vi "Get Products.vi"(8 "error in (no error) 5":errorcluster, 11 "Module Number  2":dbl=1.0) -> (0 "error out 2":errorcluster, 3 "subarray":string[](array[string]))   [LabVIEW 2015, in "Copy of Untitled Library 1.lvlib"]
uses:
  Copy of Untitled Library 1.lvlib
  Controls/Enum Constant.ctl
  <userlib>/origin_lib_main/db_interface/DB Operations Enum.ctl
  <vilib>/addons/database/_DB Variant To Data/Database Variant To Data.xnode
  <userlib>/origin_lib_main/db_interface/DB Interface.lvlib
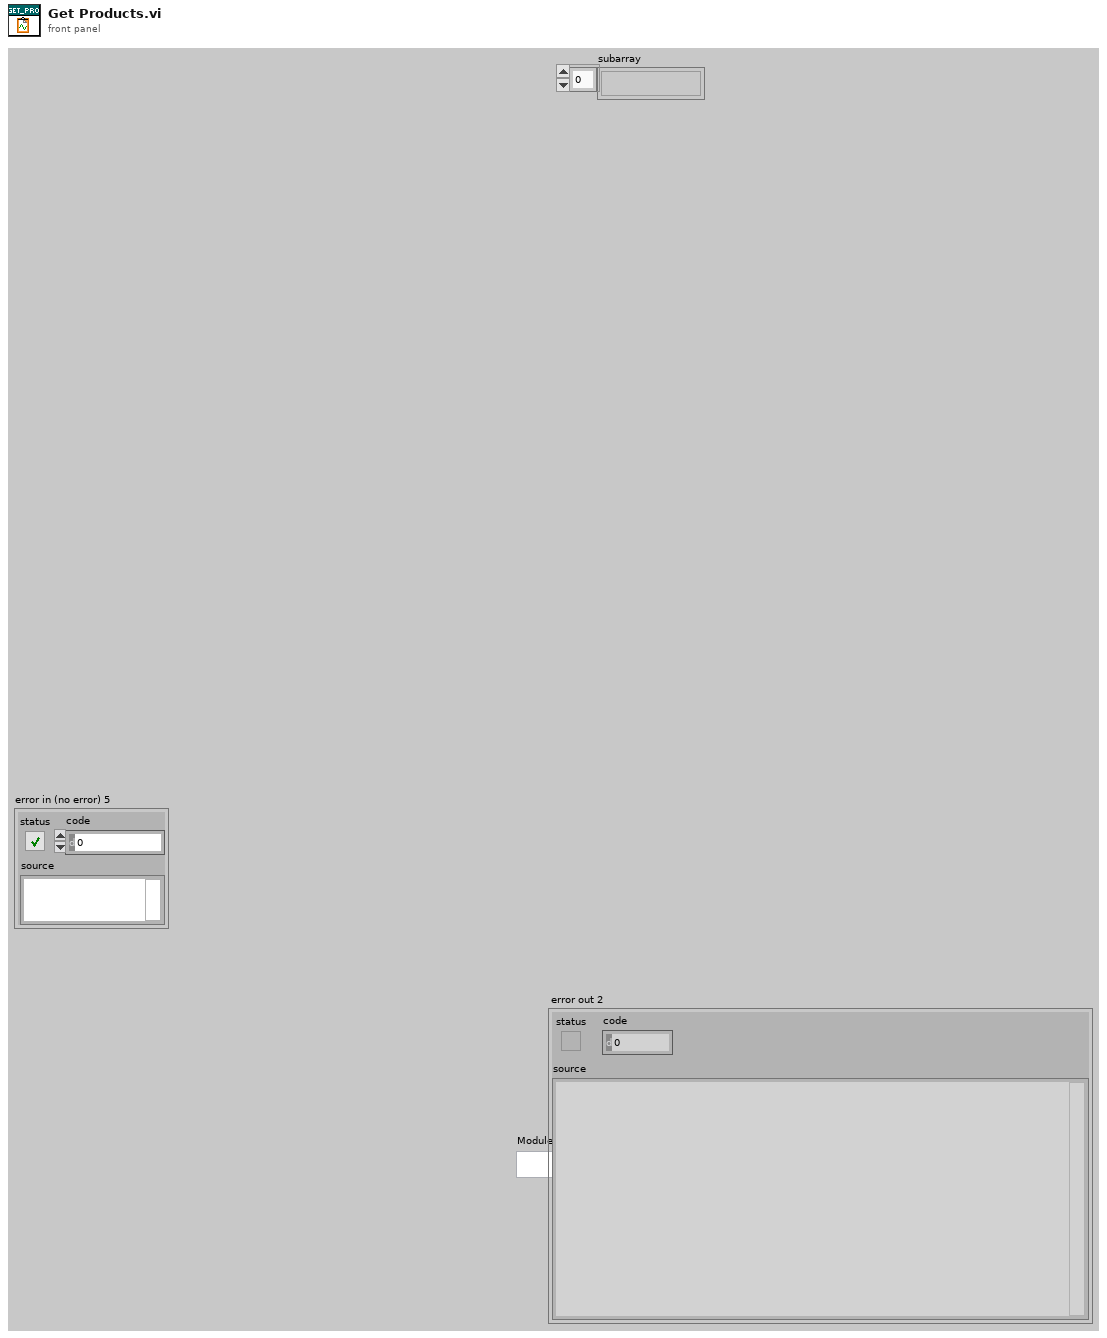
[diagram p1: front panel]
types:
  T1 = typedef "DB Interface.lvlib/DB Operations Enum.ctl" = enum16{"Select", "Update", "Insert", "Delete", "Fetch SQL Query", "Execute SQL Query", "Drop Table", "List Tables"}
  T2 = typedef "Enum Constant.ctl" = enum16{"Init", "Read", "Write"}
  T3 = typedef "FGV Data.ctl" = T4[]
  T4 = typedef "FGV Cluster Data.ctl" = cluster{"Manual/Automatic":bool, "UI Controllers ":string[], "UI Primery Key ":dbl[], "Caller Queue & MSG":T5, "Module ID":dbl, "DB Reference In":T6, "Products Columns":string[], "Cluster":cluster{"Delete Product":enum8{"Enabled", "Disabled", "Disabled and Grayed Out"}, "Add Product ":enum8{"Enabled", "Disabled", "Disabled and Grayed Out"}, "EDIT BATCH":enum8{"Enabled", "Disabled", "Disabled and Grayed Out"}, "Open Batch ":enum8{"Enabled", "Disabled", "Disabled and Grayed Out"}, "Close Batch":enum8{"Enabled", "Disabled", "Disabled and Grayed Out"}, "Delete Batch":enum8{"Enabled", "Disabled", "Disabled and Grayed Out"}, "Add Batch ":enum8{"Enabled", "Disabled", "Disabled and Grayed Out"}}}
  T5 = typedef "Queue and Caller MSG.ctl" = cluster{"Caller Queue":refnum<queue>, "Caller MSG":string}
  T6 = typedef "NI_Database_API.lvlib/Conn ObjectReference.ctl" = refnum<k1>
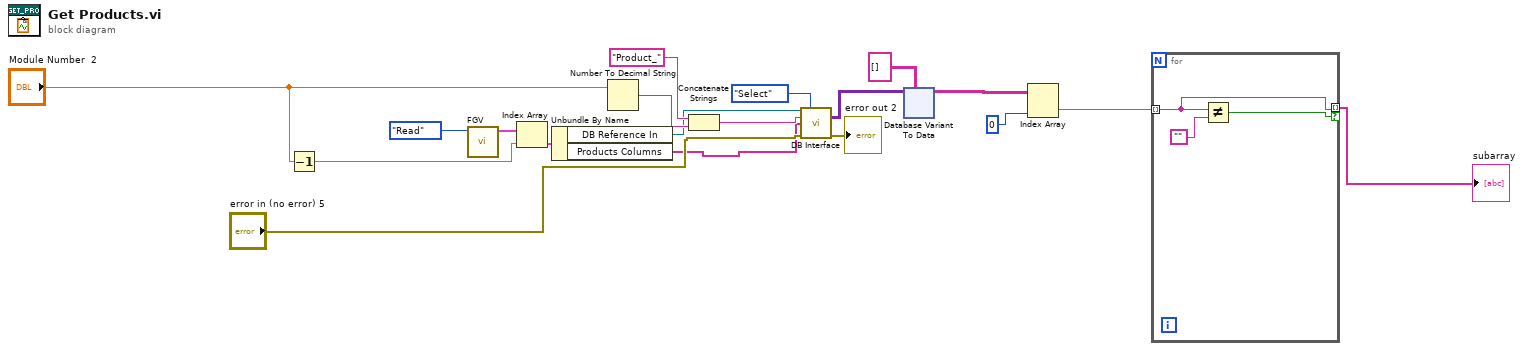
[diagram p0: block diagram]
diagram:
  n1 = Decrement(x="Module Number  2") -> (x-1=w12:dbl)
  n2 = call "FGV.vi"("Enum"=Enum_Constant."Read") -> ("Read Data"=w14:T3)  [unwired: 9 in, 1 out]
  n3 = Index Array(array=w14, index=w12) -> (element=w13:T4)
  n4 = Unbundle By Name(w13) -> ("DB Reference In"=w6:T6, "Products Columns"=w4:string[])
  n5 = Number To Decimal String(number="Module Number  2") -> (decimal integer string=w16:string)  [unwired: 1 in]
  n6 = Concatenate Strings("Product_" ("string"), w16) -> (w15:string)
  n7 = call <userlib>:"DB Interface.vi"("DB Ref In"=w6, "Operation"=DB_Operations_Enum."Select", "DB Table"=w15, "DB columns"=w4, "error in (no error)"="error in (no error) 5") -> ("data Out"=w8:variant[][], "error out"=→"error out 2":errorcluster)  [unwired: 7 in, 2 out]
  n8 = xnode "Database Variant To Data"("database variant"=w8, "type"=string[][] [] ("columns")) -> ("data"=w9:string[][])  [unwired: 1 in, 1 out]
  n9 = Index Array(array=w9, index (col)=0 ("index (row)")) -> (element=w2:string[])  [unwired: 1 in]
  n10 = for {
    tunnel: w2 -> [w20] mode=indexing
    tunnel: [w20] -> w1 mode=indexing if=w21
    n11 = Not Equal?(x=w20, y="") -> (x != y?=w21:bool)
  }
  "subarray" <- w1
